vi "Actor Core.vi"(8 "error in":errorcluster, 11 "TEC Controller in":refnum<class "TEC Controller.lvclass">) -> (0 "error out":errorcluster, 3 "Actor out":refnum<class "Actor.lvclass">)   [LabVIEW 2014, in "Humidifier Test Lib.lvlib" / "TEC Controller.lvclass"]
doc: "(<B>Filename</B>: Actor Framework.lvlib:Actor.lvclass:Actor Core.vi)\n\nReceives messages to the actor, reacts to them, and initiates any error handling that may shut the actor down.\n\nDescendant classes may override this VI to append parallel tasks for the actor to complete while it handles messages. Overrides use the Call Parent Method node."
uses:
  TEC Controller.lvclass
  <vilib>/ActorFramework/Actor/Actor.lvclass
  TEC Controller.lvclass/TEC Controller.ctl
  <vilib>/ActorFramework/Message Enqueuer/Message Enqueuer.lvclass
  Devices/Meerstetter TEC/Change Power MSG/Change Meerstetter Power.lvclass
  Devices/Meerstetter TEC/Change Power MSG/Change Meerstetter Power.lvclass/Change Meerstetter Power.ctl
  <vilib>/ActorFramework/Message Enqueuer/Message Enqueuer.lvclass/Message Enqueuer.ctl
  Devices/Alicat/Session Based/Change Setpoint Message/Change Setpoint MSG.lvclass
  Devices/Alicat/Session Based/Change Setpoint Message/Change Setpoint MSG.lvclass/Change Setpoint MSG.ctl
  Devices/Meerstetter TEC/Change Power MSG/Write Power.vi
  Devices/Alicat/Session Based/Change Setpoint Message/Write SP.vi
  <vilib>/addons/control/pid/pid.llb/PID (DBL).vi
  <vilib>/addons/control/pid/pid.llb/PID Percentage to EGU (DBL).vi
  <vilib>/ActorFramework/Message Priority Queue/Priority Enqueue.vi
  <vilib>/addons/control/pid/NI_PID_pid.lvlib
panel:
  in  "Control RH?":bool
  out "TEC":cluster{"T (degC)":dbl, "Td (degC)":dbl}
  out "Vaisala":T1
  out "Alicat":T2
  in  "RH (%)":dbl
  in  "PID":cluster{"P":dbl, "I":dbl, "D":dbl}
  in  "Q (lpm)":dbl
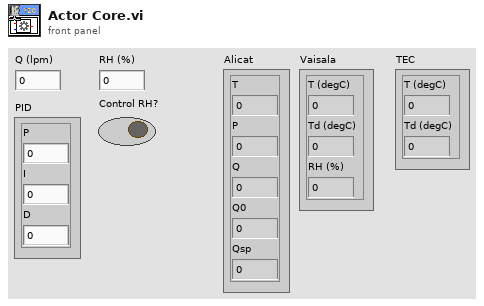
[diagram p1: front panel]
types:
  T1 = cluster{"T (degC)":dbl, "Td (degC)":dbl, "RH (%)":dbl}
  T2 = cluster{"T":dbl, "P":dbl, "Q":dbl, "Q0":dbl, "Qsp":dbl}
  T3 = cluster{"Alicat":refnum<vi>, "Vaisala":refnum<vi>, "TEC":refnum<vi>}
  T4 = cluster{"Enqueuer":refnum<class "Message Enqueuer.lvclass">, "Active":bool}
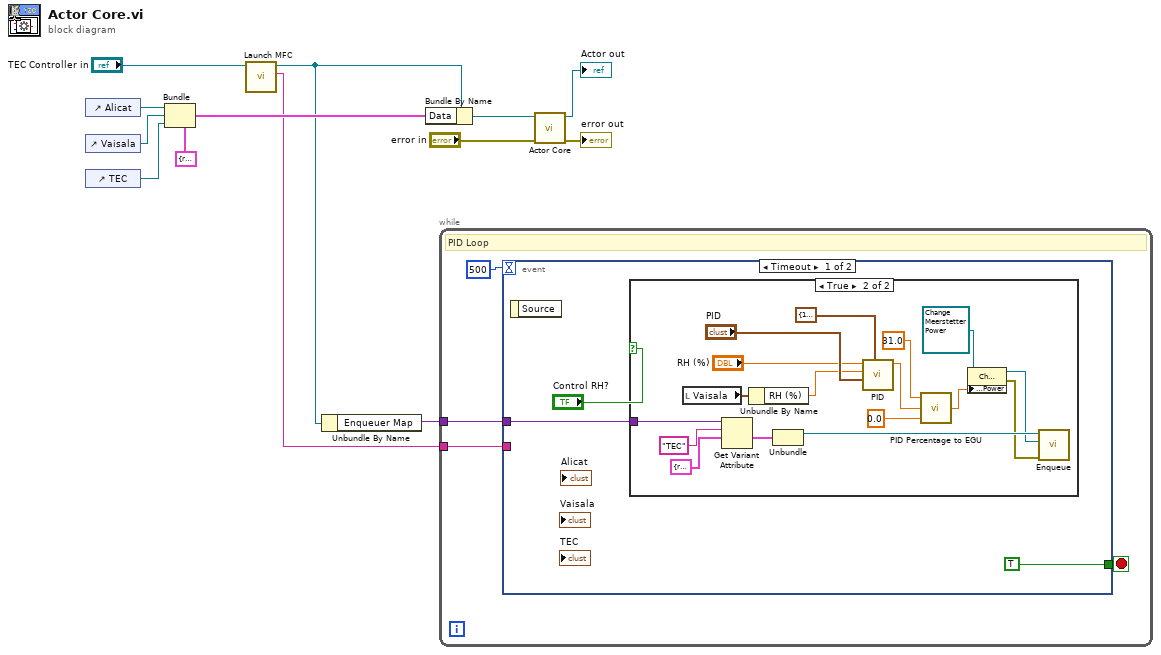
[diagram p0: block diagram]
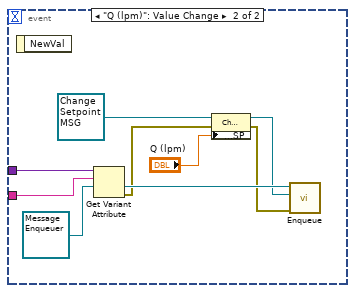
[diagram p3: hidden frame]
diagram:
  n1 = control-ref of="Alicat"() -> (w10:refnum<vi>)
  n2 = control-ref of="Vaisala"() -> (w9:refnum<vi>)
  n3 = control-ref of="TEC"() -> (w8:refnum<vi>)
  n4 = Bundle(cluster=T3 {"Alicat"=refnum, "Vaisala"=refnum, "TEC"=refnum}, "Alicat"=w10, "Vaisala"=w9, "TEC"=w8) -> (w6:T3)
  n5 = call "Launch MFC.vi"("TEC Controller in"="TEC Controller in") -> ("ID"=w1:string, "TEC Controller out"=w2:refnum<class "TEC Controller.lvclass">)  [unwired: 8 in, 1 out]
  n6 = Unbundle By Name(w2) -> ("Enqueuer Map"=w4:variant)
  n7 = Bundle By Name(cluster=w2, "Data"=w6) -> (w5:refnum<class "TEC Controller.lvclass">)
  n8 = while {
    tunnel: w4 -> [w16]
    tunnel: w1 -> [w14]
    stop <- w17 stop-if-true
    # "PID Loop"
    n9 = event shown="[0] Timeout" {
      selector: _ -> [_ _]
      dyn-events: _ -> [_ _]
      timeout: 500 -> [_ _]
      tunnel: [TRUE _] -> w17
      tunnel: w16 -> [w18 w46]
      tunnel: w14 -> [_ w39]
      event Timeout {
        n10 = event-data() -> ()  [unwired: 1 in, 1 out]
        n11 = case shown="True" "Control RH?" {
          tunnel: w18 -> [_ w32]
          frame False {
          }
          frame True {
            n12 = local read "Vaisala"() -> (w34:T1)
            n13 = Get Variant Attribute(Variant=w32, name="TEC", default value (empty Variant)=T4 {"Enqueuer"=refnum, "Active"=FALSE} ("eMap")) -> (value=w29:T4)  [unwired: 1 in, 3 out]
            n14 = Unbundle By Name(w34) -> ("RH (%)"=w33:dbl)
            n15 = Unbundle(w29) -> ("Enqueuer"=w27:refnum<class "Message Enqueuer.lvclass">)  [unwired: 1 out]
            n16 = call-poly <vilib>:"PID.vi"("output range"=cluster{"output high":dbl, "output low":dbl} {"output high"=100.0, "output low"=0.0}, "PID gains"="PID", "process variable"=w33, "setpoint"="RH (%)") -> ("output"=w24:dbl)  [unwired: 6 in, 1 out]
            n17 = call-poly <vilib>:"PID Percentage to EGU.vi"("minimum (EGU)"=0.0, "% span"=w24, "maximum (EGU)"=31.0) -> ("output (EGU)"=w21:dbl)  [unwired: 1 in]
            n18 = property class="Change Meerstetter Power"(reference=refnum<class "Change Meerstetter Power.lvclass"> refnum ("Meerstetter Lib.lvlib:Change Meerstetter Power"), "Accessors:Power"=w21) -> (reference out=w26:refnum<class "Change Meerstetter Power.lvclass">, error out=w25:errorcluster)  [unwired: 1 in]
            n19 = call <vilib>:"Enqueue.vi"("error in (no error)"=w25, "Message"=w26, "Message Enqueuer in"=w27) -> ()  [unwired: 7 in, 2 out]
          }
        }
      }
      event "Q (lpm)": Value Change {
        n20 = event-data() -> ()  [unwired: 1 in, 1 out]
        n21 = Get Variant Attribute(Variant=w46, name=w39, default value (empty Variant)=refnum<class "Message Enqueuer.lvclass"> refnum ("Self Enqueuer")) -> (value=w44:refnum<class "Message Enqueuer.lvclass">, error out=w38:errorcluster)  [unwired: 1 in, 2 out]
        n22 = property class="Change Setpoint MSG"(reference=refnum<class "Change Setpoint MSG.lvclass"> refnum ("Alicat Lib.lvlib:Change Setpoint MSG.lvclass"), error in=w38, "Accessors:SP"="Q (lpm)") -> (reference out=w41:refnum<class "Change Setpoint MSG.lvclass">, error out=w40:errorcluster)
        n23 = call <vilib>:"Enqueue.vi"("error in (no error)"=w40, "Message"=w41, "Message Enqueuer in"=w44) -> ()  [unwired: 7 in, 2 out]
      }
    }
  }
  n24 = call-parent "Actor Core.vi"("error in"="error in", "Actor in"=w5) -> ("error out"=→"error out":errorcluster, "Actor out"=→"Actor out":refnum<class "Actor.lvclass">)  [unwired: 8 in]
